vi "Read Macro Config.vi"(8 "error in (no error)":errorcluster, 11 "refnum":T2) -> (0 "error out":errorcluster, 2 "Macro Config":T1, 3 "refnum out":T2)   [LabVIEW 2020, in "MacroAssert.lvlib"]
doc: "Loads the macro defined by <B>Macro Name</B> from the config file defined by <B>refnum</B>."
uses:
  MacroAssert.lvlib
  <vilib>/ErrorRing/Error Ring.xnode
  <vilib>/Utility/config.llb/NI_LVConfig.lvlib
  <vilib>/Utility/config.llb/Read Key (String).vi
  CTLs/Macro Config V3.ctl
  <vilib>/Utility/config.llb/Read Key (U32).vi
  <vilib>/Utility/config.llb/Read Key (I32).vi
  <vilib>/Utility/error.llb/Error Cluster From Error Code.vi
  <vilib>/Utility/config.llb/Config Data RefNum.ctl
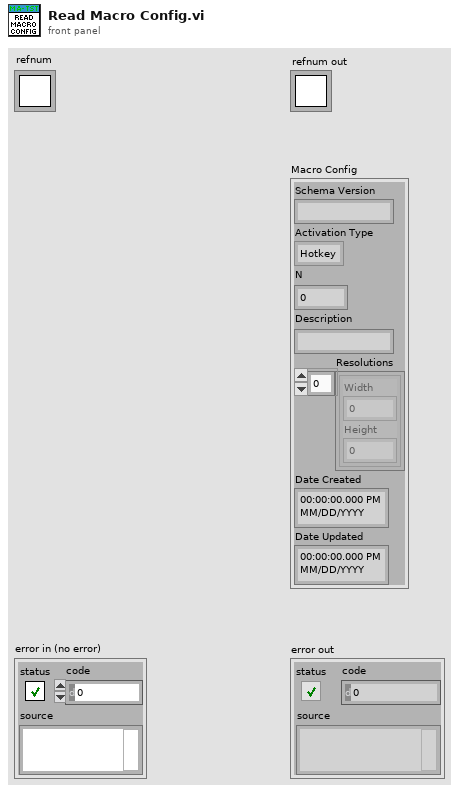
[diagram p1: front panel]
types:
  T1 = typedef "MacroAssert.lvlib/Macro Config V3.ctl" = cluster{"Schema Version":string, "Activation Type":enum32{"Hotkey", "Automatic"}, "N":i32, "Description":string, "Resolutions":cluster{"Width":i16, "Height":i16}[], "Date Created":timestamp, "Date Updated":timestamp}
  T2 = typedef "NI_LVConfig.lvlib/Config Data RefNum.ctl" = refnum<k1>
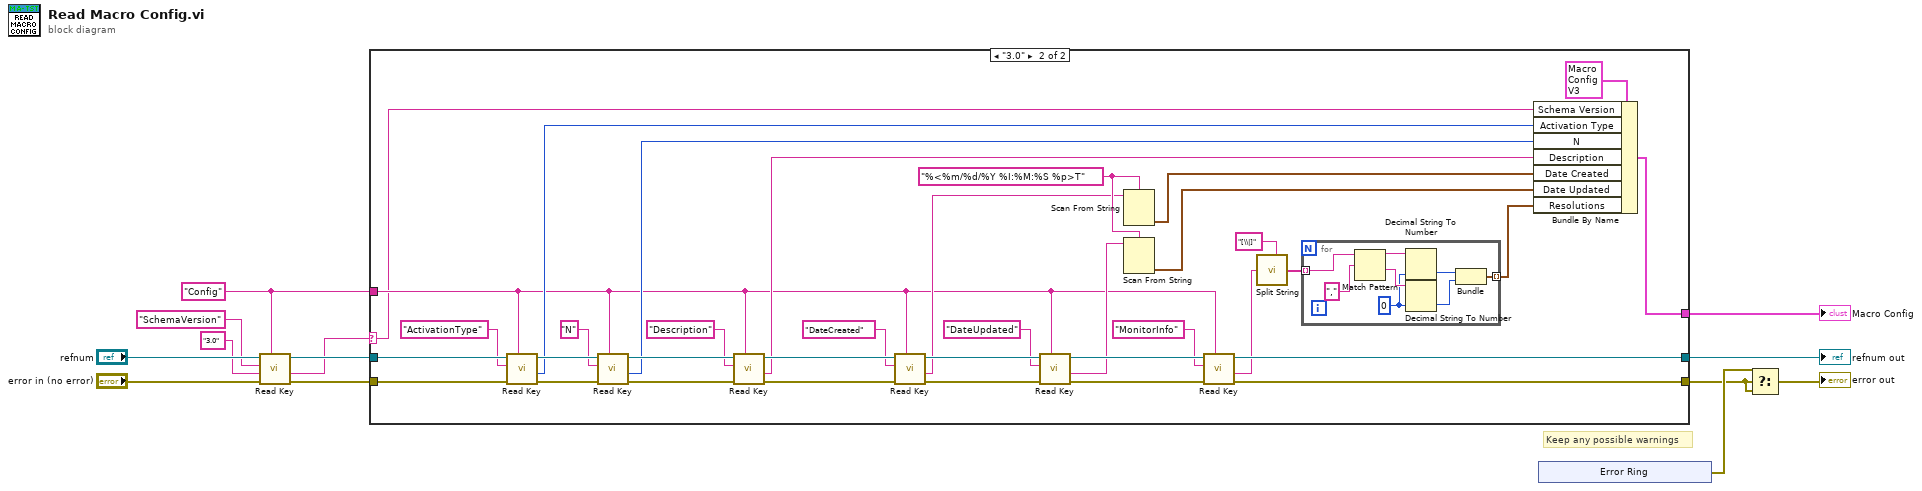
[diagram p0: block diagram]
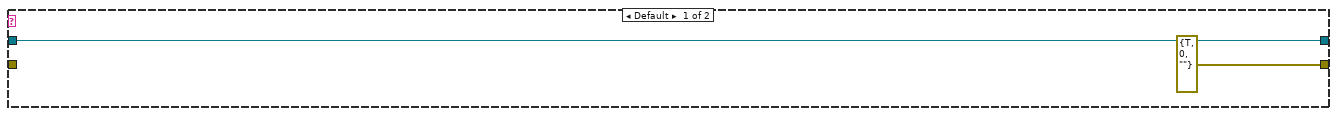
[diagram p2: hidden frame]
diagram:
  w5 = "Config" ("section")
  # "Keep any possible warnings"
  n1 = call-poly <vilib>:"Read Key.vi"("section"=w5, "error in (no error)"="error in (no error)", "default value"="3.0", "key"="SchemaVersion", "refnum"="refnum") -> ("error out"=w9:errorcluster, "value"=w6:string, "refnum out"=w10:T2)  [unwired: 3 in, 1 out]
  n2 = case shown="\"3.0\"" w6 {
    selector: w6 -> [_ w16]
    tunnel: w10 -> [w15 w51]
    tunnel: [w15 w23] -> w3
    tunnel: w9 -> [_ w44]
    tunnel: w5 -> [_ w17]
    tunnel: [errorcluster {"status"=TRUE, "code"=0, "source"=""} ("error out") w22] -> w2
    tunnel: [_ w43] -> w1
    frame Default {
    }
    frame "3.0" {
      w32 = "%<%m/%d/%Y %I:%M:%S %p>T" ("format string")
      n3 = call-poly <vilib>:"Read Key.vi"("section"=w17, "error in (no error)"=w44, "key"="ActivationType", "refnum"=w51) -> ("error out"=w40:errorcluster, "value"=w35:u32, "refnum out"=w50:T2)  [unwired: 4 in, 1 out]
      n4 = call-poly <vilib>:"Read Key.vi"("section"=w17, "error in (no error)"=w40, "key"="N", "refnum"=w50) -> ("error out"=w38:errorcluster, "value"=w34:i32, "refnum out"=w49:T2)  [unwired: 4 in, 1 out]
      n5 = call-poly <vilib>:"Read Key.vi"("section"=w17, "error in (no error)"=w38, "key"="Description", "refnum"=w49) -> ("error out"=w36:errorcluster, "value"=w33:string, "refnum out"=w48:T2)  [unwired: 4 in, 1 out]
      n6 = call-poly <vilib>:"Read Key.vi"("section"=w17, "error in (no error)"=w36, "key"="DateCreated", "refnum"=w48) -> ("error out"=w28:errorcluster, "value"=w26:string, "refnum out"=w47:T2)  [unwired: 4 in, 1 out]
      n7 = call-poly <vilib>:"Read Key.vi"("section"=w17, "error in (no error)"=w28, "key"="DateUpdated", "refnum"=w47) -> ("error out"=w24:errorcluster, "value"=w25:string, "refnum out"=w46:T2)  [unwired: 4 in, 1 out]
      n8 = Scan From String(format string=w32, input string=w26) -> (output 1=w31:timestamp)  [unwired: 3 in, 3 out]
      n9 = Scan From String(format string=w32, input string=w25) -> (output 1=w30:timestamp)  [unwired: 3 in, 3 out]
      n10 = call-poly <vilib>:"Read Key.vi"("section"=w17, "error in (no error)"=w24, "key"="MonitorInfo", "refnum"=w46) -> ("error out"=w22:errorcluster, "value"=w19:string, "refnum out"=w23:T2)  [unwired: 4 in, 1 out]
      n11 = call <vilib>:"Split String.vi"("Split Pattern"="[\\|]", "Input String"=w19) -> ("Split String"=w21:string[])  [unwired: 5 in]
      n12 = for {
        tunnel: w21 -> [w59] mode=indexing
        tunnel: [w53] -> w18 mode=indexing
        w52 = i16 0 ("default (0 I32)")
        n13 = Match Pattern(string=w59, regular expression=",") -> (before substring=w57:string, after substring=w56:string)  [unwired: 1 in, 2 out]
        n14 = Decimal String To Number(string=w57, default (0L)=w52) -> (number=w55:i16)  [unwired: 1 in, 1 out]
        n15 = Decimal String To Number(string=w56, default (0L)=w52) -> (number=w54:i16)  [unwired: 1 in, 1 out]
        n16 = Bundle(w55, w54) -> (w53:cluster{i16, i16})  [unwired: 1 in]
      }
      n17 = Bundle By Name(cluster=T1 {"Schema Version"="", "Activation Type"=enum."Hotkey", "N"=0, "Description"="", "Resolutions"=[], "Date Created"=timestamp(0 s since 1904-01-01), "Date Updated"=timestamp(0 s since 1904-01-01)} ("Macro Config"), "Schema Version"=w16, "Activation Type"=w35, "N"=w34, "Description"=w33, "Date Created"=w31, "Date Updated"=w30, "Resolutions"=w18) -> (w43:T1)
    }
  }
  "refnum out" <- w3
  "Macro Config" <- w1
  n18 = xnode "Error Ring"() -> ("error out"=w12:errorcluster)
  n19 = Select(t=w12, s=w2, f=w2) -> (s? t:f=→"error out":errorcluster)
